vi "Database Main.vi"(1 "Group By":string, 4 "Order By":string, 5 "DB Name/Path":string="framework", 6 "Option":T1, 7 "Where":string, 8 "error in (no error)":errorcluster, 9 "Column Values":string[][](array[string])=[["1", "\"A\"", "\"C\""]], 10 "Column Name":string[](array[string]), 11 "table Name/Query":string="sys_station_config") -> (0 "error out":errorcluster, 2 "Count":i32, 3 "Data":string[][](array[string]))   [LabVIEW 2020]
uses:
  Controls/DB Options.ctl
  D:/Labview/Auto Run Screen/Source Code/Database/Support/dbquery.dll
  Support/dbquery.dll
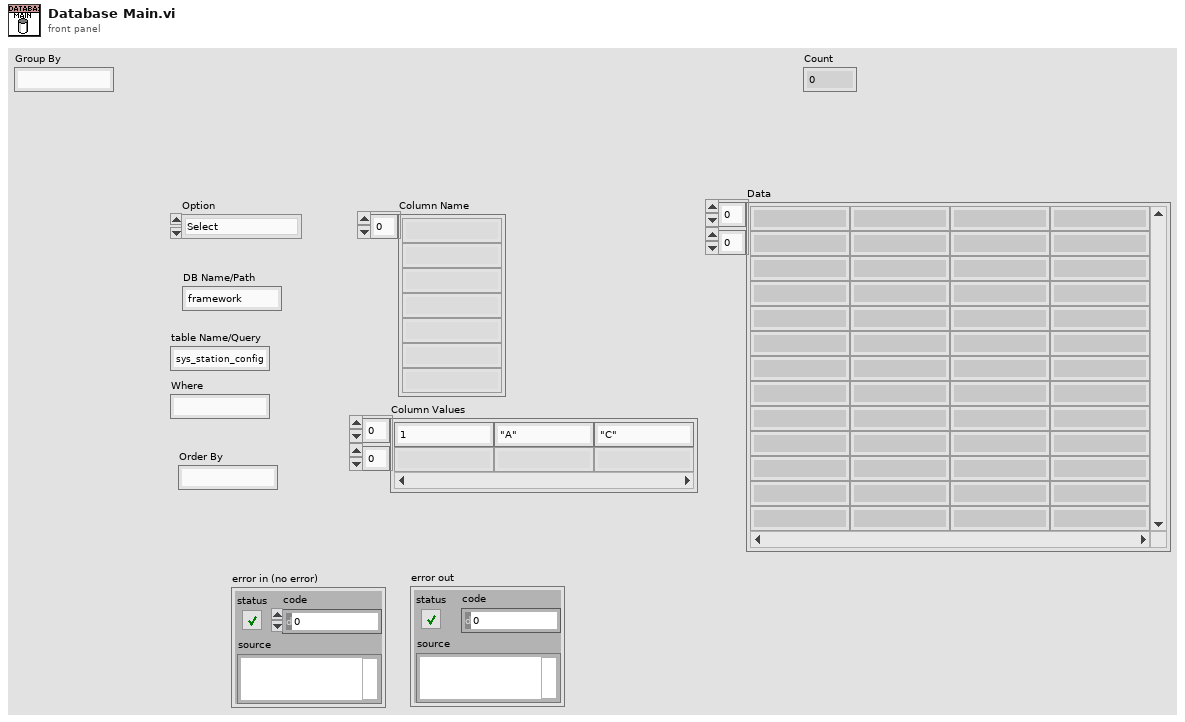
[diagram p1: front panel]
types:
  T1 = typedef "DB Options.ctl" = enum16{"Select", "Execute", "Special Q", "Insert", "Update", "Delete", "Open", "Close"}
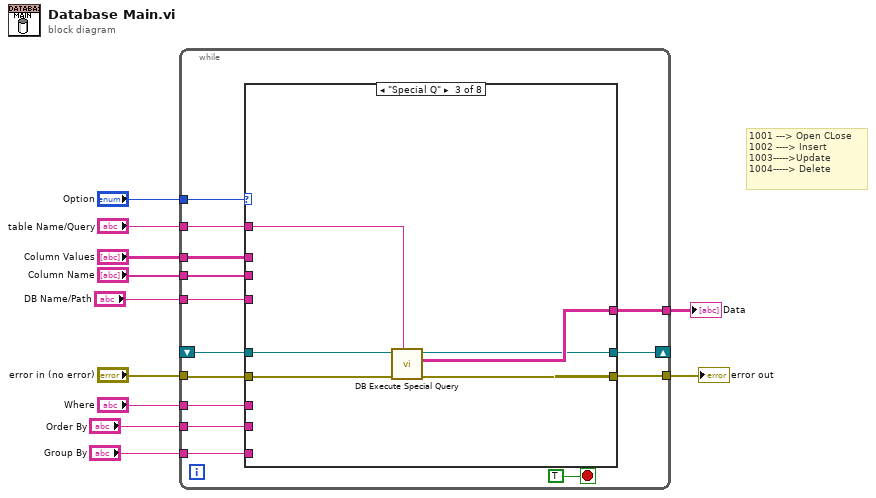
[diagram p0: block diagram]
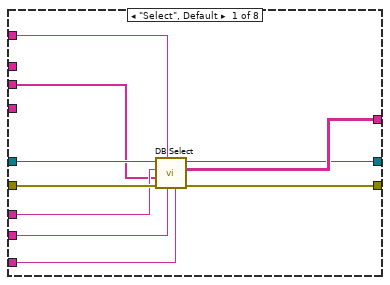
[diagram p2: hidden frame]
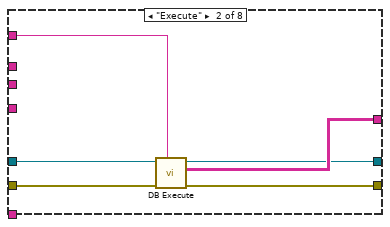
[diagram p3: hidden frame]
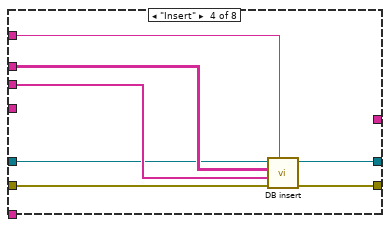
[diagram p4: hidden frame]
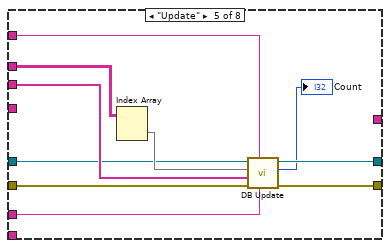
[diagram p5: hidden frame]
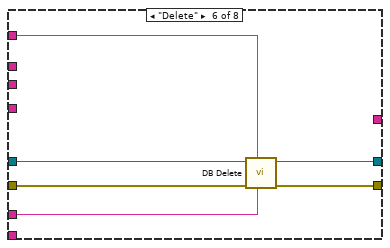
[diagram p6: hidden frame]
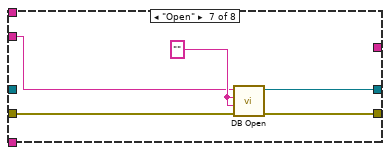
[diagram p7: hidden frame]
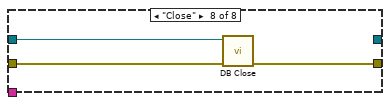
[diagram p8: hidden frame]
diagram:
  # "1001 ---> Open CLose\n1002 ----> Insert\n1003----->Update\n1004-----> Delete"
  n1 = while {
    tunnel: [w24] -> w11
    tunnel: "error in (no error)" -> [w23]
    tunnel: "Option" -> [w22]
    tunnel: [w21] -> w8
    shift-right: [w20] -> _
    shift-left: _ -> [w19]
    tunnel: "table Name/Query" -> [w18]
    tunnel: "Where" -> [w17]
    tunnel: "Column Name" -> [w16]
    tunnel: "Column Values" -> [w15]
    tunnel: "Order By" -> [w14]
    tunnel: "DB Name/Path" -> [w13]
    tunnel: "Group By" -> [w12]
    stop <- TRUE stop-if-true
    n2 = case shown="\"Special Q\"" w22 {
      tunnel: w23 -> [w33 w39 w45 w54 w64 w70 w75 w77]
      tunnel: [w32 w38 w44 w53 w63 w69 w74 w78] -> w21
      tunnel: [w34 w40 w46 w52 w62 w68 w73 _] -> w20
      tunnel: w18 -> [w31 w37 w43 w51 w61 w67 _ _]
      tunnel: w16 -> [w28 _ _ w50 w60 _ _ _]
      tunnel: [w35 w41 w47 _ _ _ _ _] -> w24
      tunnel: w17 -> [w29 _ _ _ w59 w66 _ _]
      tunnel: w19 -> [w30 w36 w42 w48 w56 w65 _ w76]
      tunnel: w15 -> [_ _ _ w49 w58 _ _ _]
      tunnel: w14 -> [w27 _ _ _ _ _ _ _]
      tunnel: w13 -> [_ _ _ _ _ _ w71 _]
      tunnel: w12 -> [w26 _ _ _ _ _ _ _]
      frame "Select", Default {
        n3 = call "DB Select.vi"("Group By"=w26, "Orderby"=w27, "table Name"=w31, "error in (no error)"=w33, "Column Name"=w28, "Where Condition"=w29, "Db Reference"=w30) -> ("error out"=w32:errorcluster, "Data"=w35:string[][], "Db Reference"=w34:refnum<k24>)  [unwired: 2 in]
      }
      frame "Execute" {
        n4 = call "DB Execute.vi"("table Name"=w37, "error in (no error)"=w39, "Db Reference"=w36) -> ("error out"=w38:errorcluster, "Data"=w41:string[][], "Db Reference"=w40:refnum<k24>)  [unwired: 6 in]
      }
      frame "Special Q" {
        n5 = call "DB Execute Special Query.vi"("table Name"=w43, "error in (no error)"=w45, "Db Reference"=w42) -> ("error out"=w44:errorcluster, "Data"=w47:string[][], "Db Reference"=w46:refnum<k24>)  [unwired: 6 in]
      }
      frame "Insert" {
        n6 = call "DB insert.vi"("table Name"=w51, "error in (no error)"=w54, "Column Name"=w50, "Column Values"=w49, "Db Reference"=w48) -> ("error out"=w53:errorcluster, "Db Reference"=w52:refnum<k24>)  [unwired: 5 in]
      }
      frame "Update" {
        n7 = Index Array(array=w58) -> (element=w57:string[])  [unwired: 2 in]
        n8 = call "DB Update.vi"("Where"=w59, "table Name"=w61, "error in (no error)"=w64, "Column Name"=w60, "Column Values"=w57, "Db Reference"=w56) -> ("error out"=w63:errorcluster, "data"=→"Count":i32, "Db Reference"=w62:refnum<k24>)  [unwired: 3 in]
      }
      frame "Delete" {
        n9 = call "DB Delete.vi"("Where"=w66, "table Name"=w67, "error in (no error)"=w70, "Db Reference"=w65) -> ("error out"=w69:errorcluster, "Db Reference"=w68:refnum<k24>)  [unwired: 6 in]
      }
      frame "Open" {
        w72 = "" ("UserID")
        n10 = call "DB Open.vi"("error in (no error)"=w75, "Password"=w72, "UserID"=w72, "dbpath"=w71) -> ("error out"=w74:errorcluster, "Db Reference Out"=w73:refnum<k24>)  [unwired: 6 in]
      }
      frame "Close" {
        n11 = call "DB Close.vi"("error in (no error)"=w77, "Db Reference"=w76) -> ("error out"=w78:errorcluster)  [unwired: 9 in]
      }
    }
  }
  "Data" <- w11
  "error out" <- w8
